vi "Read Controllers.vi"   [LabVIEW 2014]
uses:
  Begin/Global RefNums.vi
  <vilib>/Rock Robotics/WPI/Joystick/WPI_JoystickGetSetRefNum.vi
  Begin/Global Variables.vi
types:
  T1 = typedef "WPI_JoystickDevRef.ctl" = cluster{"Device":T2}
  T2 = typedef "WPI_JoystickDeviceEnum.ctl" = enum16{"USB 0", "USB 1", "USB 2", "USB 3", "USB 4", "USB 5"}
  T3 = cluster{"Axes[0]":dbl, "Axes[1]":dbl, "Axes[2]":dbl, "Axes[3]":dbl, "Axes[4]":dbl, "Axes[5]":dbl, "Axes[6]":dbl, "Axes[7]":dbl, "Axes[8]":dbl}
  T4 = cluster{"Buttons[0]":bool, "Buttons[1]":bool, "Buttons[2]":bool, "Buttons[3]":bool, "Buttons[4]":bool, "Buttons[5]":bool, "Buttons[6]":bool, "Buttons[7]":bool, "Buttons[8]":bool}
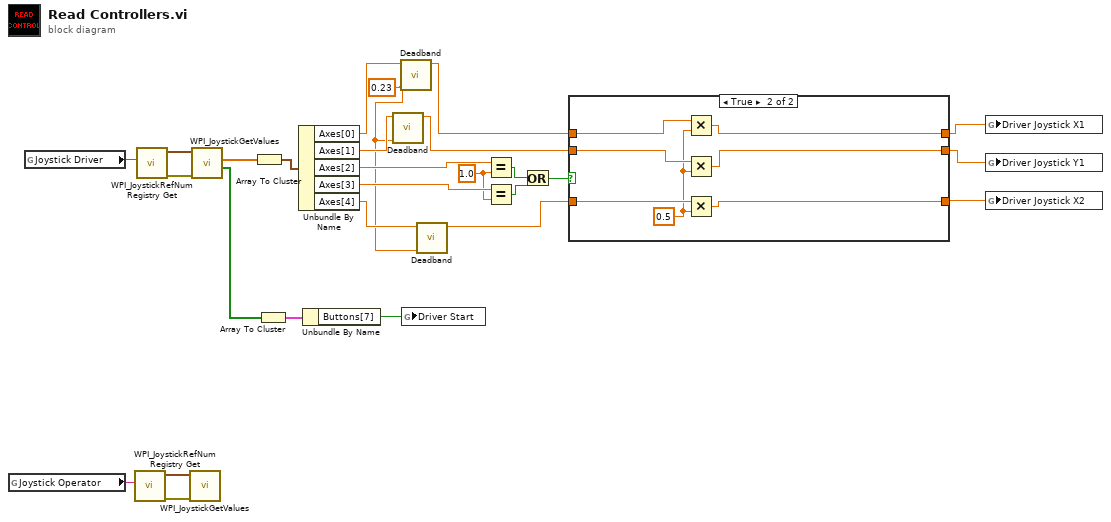
[diagram p0: block diagram]
diagram:
  w1 = 0.23 ("Value to Deadband (default of 0.1)")
  w11 = 1.0 ("y")
  n1 = global read "Global RefNums.vi" "Joystick Operator"() -> (w22:string)
  n2 = global read "Global RefNums.vi" "Joystick Driver"() -> (w27:string)
  n3 = call <vilib>:"WPI_JoystickRefNum Registry Get.vi"("refnum name"=w22) -> ("error out"=w24:errorcluster, "JoystickDevRef"=w23:T1)  [unwired: 9 in]
  n4 = call <vilib>:"WPI_JoystickRefNum Registry Get.vi"("refnum name"=w27) -> ("error out"=w25:errorcluster, "JoystickDevRef"=w26:T1)  [unwired: 9 in]
  n5 = call <vilib>:"WPI_JoystickGetValues.vi"("error in (no error)"=w24, "JoystickDevRef"=w23) -> ()  [unwired: 5 in, 5 out]
  n6 = call <vilib>:"WPI_JoystickGetValues.vi"("error in (no error)"=w25, "JoystickDevRef"=w26) -> ("Buttons"=w10:bool[], "Axes"=w21:dbl[])  [unwired: 5 in, 3 out]
  n7 = Array To Cluster(array=w21) -> (cluster=w20:T3)
  n8 = Array To Cluster(array=w10) -> (cluster=w9:T4)
  n9 = Unbundle By Name(w20) -> ("Axes[0]"=w7:dbl, "Axes[1]"=w5:dbl, "Axes[2]"=w16:dbl, "Axes[3]"=w12:dbl, "Axes[4]"=w3:dbl)
  n10 = Unbundle By Name(w9) -> ("Buttons[7]"=w8:bool)
  n11 = call "Deadband.vi"("Value to Deadband (default of 0.1)"=w1, "Value"=w5) -> ("Deadbanded Value"=w4:dbl)  [unwired: 9 in]
  n12 = call "Deadband.vi"("Value to Deadband (default of 0.1)"=w1, "Value"=w7) -> ("Deadbanded Value"=w6:dbl)  [unwired: 9 in]
  n13 = global write "Global Variables.vi" "Driver Start"(w8) -> ()
  n14 = call "Deadband.vi"("Value to Deadband (default of 0.1)"=w1, "Value"=w3) -> ("Deadbanded Value"=w2:dbl)  [unwired: 9 in]
  n15 = Equal?(x=w16, y=w11) -> (x = y?=w14:bool)
  n16 = Equal?(x=w12, y=w11) -> (x = y?=w13:bool)
  n17 = Or(x=w14, y=w13) -> (x .or. y?=w15:bool)
  n18 = case shown="True" w15 {
    tunnel: w6 -> [w28 w37]
    tunnel: w4 -> [w29 w36]
    tunnel: w2 -> [w30 w35]
    tunnel: [w30 w31] -> w18
    tunnel: [w29 w32] -> w17
    tunnel: [w28 w33] -> w19
    frame False {
    }
    frame True {
      w34 = 0.5 ("y")
      n19 = Multiply(x=w37, y=w34) -> (x*y=w33:dbl)
      n20 = Multiply(x=w36, y=w34) -> (x*y=w32:dbl)
      n21 = Multiply(x=w35, y=w34) -> (x*y=w31:dbl)
    }
  }
  n22 = global write "Global Variables.vi" "Driver Joystick X1"(w19) -> ()
  n23 = global write "Global Variables.vi" "Driver Joystick Y1"(w17) -> ()
  n24 = global write "Global Variables.vi" "Driver Joystick X2"(w18) -> ()
